vi "_r_n.vi"() -> (3 "command":string)   [LabVIEW 2023, in "ELTA.lvlib"]
uses:
  ELTA.lvlib
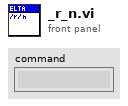
[diagram p1: front panel]
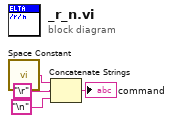
[diagram p0: block diagram]
diagram:
  n1 = call <vilib>:"Space Constant.vi"() -> ("String"=w4:string)
  n2 = Concatenate Strings(w4, "\r", "\n") -> (→"command":string)
